vi "Spreadsheet Array to Column Map.vi"(11 "array":string[][](array[string])) -> (3 "map":map{string, string[]}(c390))   [LabVIEW 2020, in "Logging Loopback.lvclass"]
uses:
  Logging Loopback.lvclass
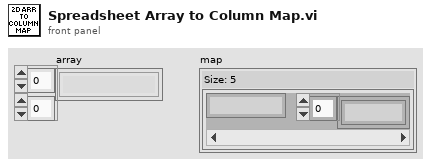
[diagram p1: front panel]
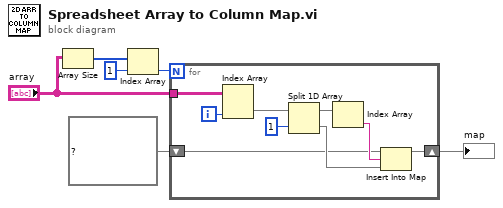
[diagram p0: block diagram]
diagram:
  n1 = Array Size(array="array") -> (size(s)=w6:i32[])
  n2 = Index Array(array=w6, index=1) -> (element=w1:i32)
  n3 = for {
    N: w1 -> [_]
    tunnel: "array" -> [w15]
    shift-right: [w8] -> w2
    shift-left: map{string, string[]} {} ("map") -> [w9]
    i -> [w14]
    n4 = Index Array(array=w15, index (col)=w14) -> (element=w7:string[])  [unwired: 1 in]
    n5 = Split 1D Array(array=w7, index=1) -> (first subarray=w12:string[], second subarray=w10:string[])
    n6 = Index Array(array=w12) -> (element=w11:string)  [unwired: 1 in]
    n7 = Insert Into Map(map in=w9, key=w11, value=w10) -> (map out=w8:map{string, string[]})  [unwired: 2 out]
  }
  "map" <- w2
